vi "configureImageTiming.vi"(6 "Timeout":dbl, 8 "error in (no error)":errorcluster, 9 "Shift Speed":T1, 10 "Timing":T2, 11 "CameraAcquisitor in":refnum<class "CameraAcquisitor.lvclass">) -> (0 "error out":errorcluster, 3 "CameraAcquisitor out":refnum<class "CameraAcquisitor.lvclass">)   [LabVIEW 2009, in "Hardware.lvlib" / "Channels.lvlib" / "CameraAcquisitor.lvclass"]
uses:
  CameraAcquisitor.lvclass
  CameraAcquisitor.lvclass/CameraAcquisitor.ctl
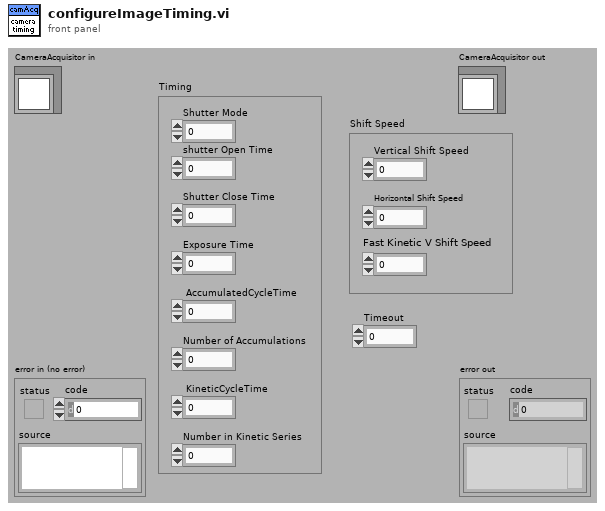
[diagram p1: front panel]
types:
  T1 = cluster{"Vertical Shift Speed":dbl, "Horizontal Shift Speed":dbl, "Fast Kinetic V Shift Speed":dbl}
  T2 = cluster{"shutter Open Time":dbl, "Shutter Close Time":dbl, "Exposure Time":dbl, " AccumulatedCycleTime":dbl, " KineticCycleTime":dbl, "Number of Accumulations":dbl, "Number in Kinetic Series ":dbl, "Shutter Mode":dbl}
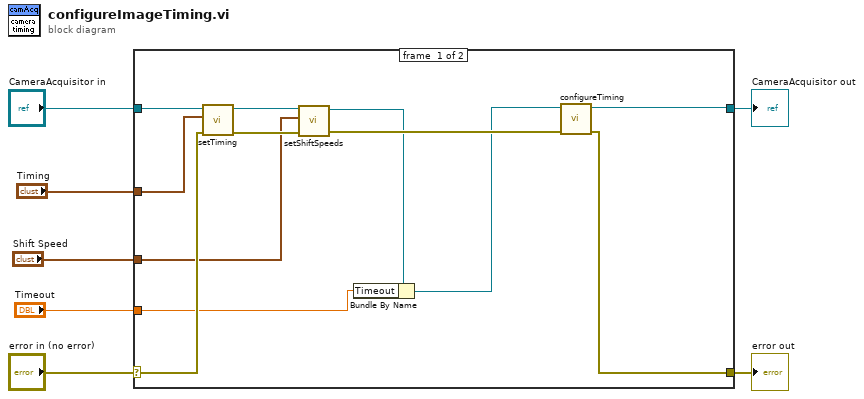
[diagram p0: block diagram]
diagram:
  n1 = case shown="No Error" "error in (no error)" {
    selector: "error in (no error)" -> [w18 w21]
    tunnel: [w13 w21] -> w6
    tunnel: [w12 w20] -> w4
    tunnel: "CameraAcquisitor in" -> [w19 w20]
    tunnel: "Timing" -> [w11 _]
    tunnel: "Shift Speed" -> [w15 _]
    tunnel: "Timeout" -> [w8 _]
    frame #0 {
      n2 = call-dynamic "setTiming.vi"("error in (no error)"=w18, "Timing"=w11, "CameraAcquisitor.lvclass in"=w19) -> ("error out"=w16:errorcluster, "CameraAcquisitor.lvclass out"=w17:refnum<class "CameraAcquisitor.lvclass">)  [unwired: 7 in]
      n3 = call-dynamic "setShiftSpeeds.vi"("error in (no error)"=w16, "Shift Speed"=w15, "CameraAcquisitor.lvclass in"=w17) -> ("error out"=w14:errorcluster, "CameraAcquisitor.lvclass out"=w10:refnum<class "CameraAcquisitor.lvclass">)  [unwired: 7 in]
      n4 = Bundle By Name(cluster=w10, "Timeout"=w8) -> (w9:refnum<class "CameraAcquisitor.lvclass">)
      n5 = call-dynamic "configureTiming.vi"("error in (no error)"=w14, "CameraAcquisitor in"=w9) -> ("error out"=w13:errorcluster, "CameraAcquisitor out"=w12:refnum<class "CameraAcquisitor.lvclass">)  [unwired: 8 in]
    }
    frame #1 {
    }
  }
  "error out" <- w6
  "CameraAcquisitor out" <- w4
